vi "Add Channel Name.vi"(8 "error in (no error)":errorcluster, 9 "Channel Names":string[](array[string]), 10 "Table Name":string, 11 "Abstruct Data Type in":refnum<class "Abstruct Data Type.lvclass">) -> (0 "error out":errorcluster, 3 "Abstruct Data Type out":refnum<class "Abstruct Data Type.lvclass">)   [LabVIEW 2020, in "Abstruct Data Type.lvclass"]
uses:
  Abstruct Data Type.lvclass
  Abstruct Data Type.lvclass/Abstruct Data Type.ctl
  Data List/Data List.lvclass/Data List.ctl
  Data List/Data List.lvclass
  Data List/Accessors/Read Table Name.vi
  2984df62-0dc3-48fe-846c-8cf793447fad.vi
  Data List/Accessors/Write Table Name.vi
  Data List/Accessors/Write Channels Names.vi
  Data List/Accessors/Write File Path.vi
  Data List/Accessors/Read Channels Names.vi
  Accessors/Read Table Infor.vi
  Accessors/Read File Path.vi
  Accessors/Write Table Infor.vi
  2984df62-0dc3-48fe-846c-8cf793447fad.vi/d4db2432-cc9c-482c-8957-dac855435ef6.vi
  2984df62-0dc3-48fe-846c-8cf793447fad.vi/86fbf154-bd7b-49a2-8ab2-a837b2a95f24.vi
  2984df62-0dc3-48fe-846c-8cf793447fad.vi/3b95b01e-1ec2-4565-bcd9-7606a5281010.vi
  2984df62-0dc3-48fe-846c-8cf793447fad.vi/96a08935-737a-44b2-979c-a81d56408f7e.vi
  2984df62-0dc3-48fe-846c-8cf793447fad.vi/d4db2432-cc9c-482c-8957-dac855435ef6.vi/6eaecd13-6e48-4772-a921-b51ebdf84d88.vi
  2984df62-0dc3-48fe-846c-8cf793447fad.vi/d4db2432-cc9c-482c-8957-dac855435ef6.vi/d2d5f2b7-06f4-47f6-971c-049c3fdbb653.vi
  2984df62-0dc3-48fe-846c-8cf793447fad.vi/3b95b01e-1ec2-4565-bcd9-7606a5281010.vi/6eaecd13-6e48-4772-a921-b51ebdf84d88.vi
  2984df62-0dc3-48fe-846c-8cf793447fad.vi/3b95b01e-1ec2-4565-bcd9-7606a5281010.vi/d2d5f2b7-06f4-47f6-971c-049c3fdbb653.vi
  2984df62-0dc3-48fe-846c-8cf793447fad.vi/96a08935-737a-44b2-979c-a81d56408f7e.vi/6eaecd13-6e48-4772-a921-b51ebdf84d88.vi
  2984df62-0dc3-48fe-846c-8cf793447fad.vi/96a08935-737a-44b2-979c-a81d56408f7e.vi/d2d5f2b7-06f4-47f6-971c-049c3fdbb653.vi
  <vilib>/Comparison/Less/Less Functor/Less Functor.lvclass
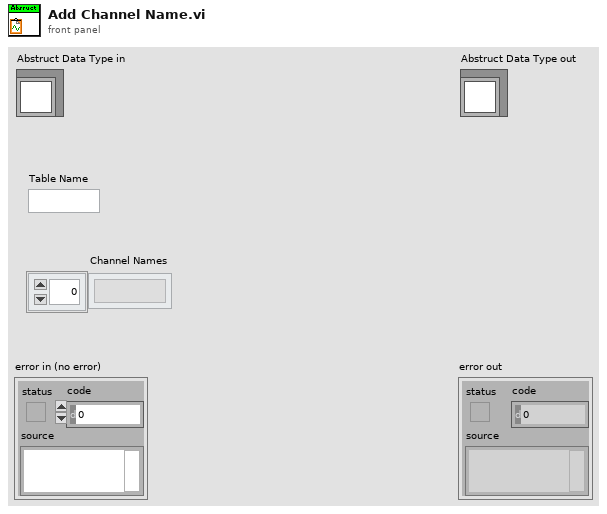
[diagram p1: front panel]
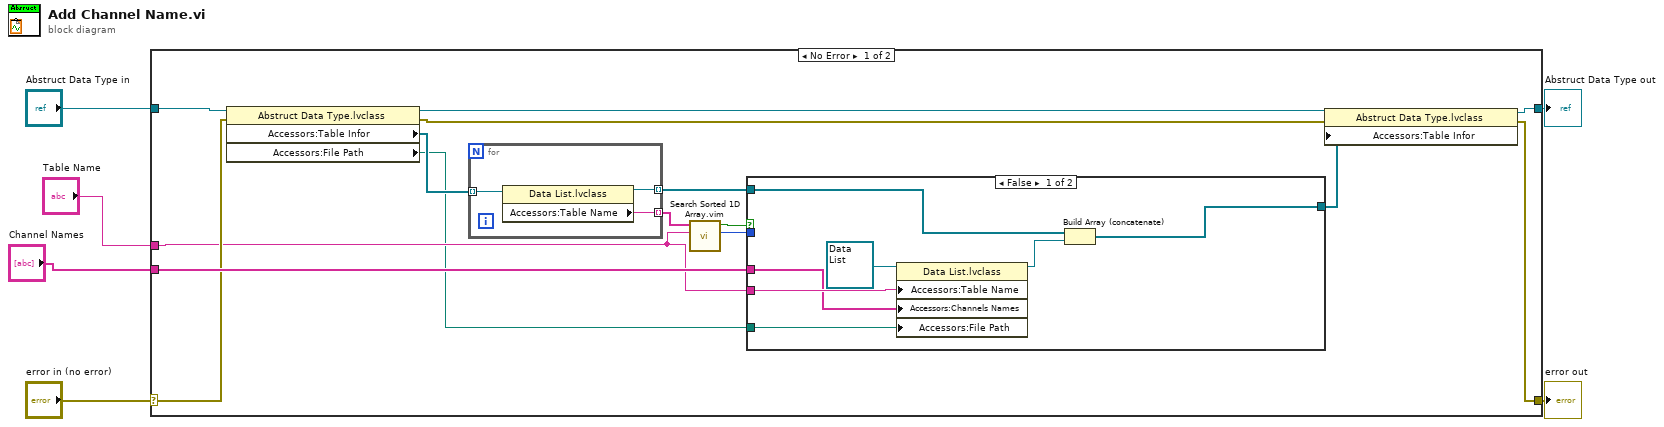
[diagram p0: block diagram]
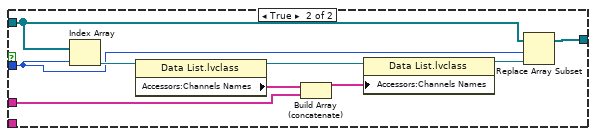
[diagram p2: hidden frame]
diagram:
  n1 = case shown="No Error" "error in (no error)" {
    selector: "error in (no error)" -> [w9 w42]
    tunnel: [w11 w42] -> w5
    tunnel: [w12 w41] -> w3
    tunnel: "Abstruct Data Type in" -> [w21 w41]
    tunnel: "Table Name" -> [w8 _]
    tunnel: "Channel Names" -> [w15 _]
    frame No Error {
      n2 = property class="Abstruct Data Type.lvclass"(reference=w21, error in=w9) -> (reference out=w13:refnum<class "Abstruct Data Type.lvclass">, error out=w10:errorcluster, "Accessors:Table Infor"=w20:refnum<class "Data List.lvclass">[], "Accessors:File Path"=w7:path)
      n3 = for {
        tunnel: w20 -> [w40] mode=indexing
        tunnel: [w39] -> w16 mode=indexing
        tunnel: [w38] -> w19 mode=indexing
        n4 = property class="Data List.lvclass"(reference=w40) -> (reference out=w39:refnum<class "Data List.lvclass">, "Accessors:Table Name"=w38:string)  [unwired: 1 in, 1 out]
      }
      n5 = call "Search Sorted 1D Array.vim"("element"=w8, "sorted 1D array"=w19) -> ("nearest index"=w17:i32, "found?"=w18:bool)  [unwired: 8 in]
      n6 = case shown="False" w18 {
        tunnel: w17 -> [_ w31]
        tunnel: w16 -> [w28 w32]
        tunnel: w15 -> [w23 w34]
        tunnel: [w25 w29] -> w14
        tunnel: w8 -> [w24 _]
        tunnel: w7 -> [w22 _]
        frame False {
          n7 = property class="Data List.lvclass"(reference=refnum<class "Data List.lvclass"> refnum ("Data List.lvclass"), "Accessors:Table Name"=w24, "Accessors:Channels Names"=w23, "Accessors:File Path"=w22) -> (reference out=w26:refnum<class "Data List.lvclass">)  [unwired: 1 in, 1 out]
          n8 = Build Array (concatenate)(w28, w26) -> (w25:refnum<class "Data List.lvclass">[])
        }
        frame True {
          n9 = Index Array(array=w32, index=w31) -> (element=w37:refnum<class "Data List.lvclass">)
          n10 = property class="Data List.lvclass"(reference=w37) -> (reference out=w33:refnum<class "Data List.lvclass">, "Accessors:Channels Names"=w36:string[])  [unwired: 1 in, 1 out]
          n11 = Build Array (concatenate)(w36, w34) -> (w35:string[])
          n12 = property class="Data List.lvclass"(reference=w33, "Accessors:Channels Names"=w35) -> (reference out=w30:refnum<class "Data List.lvclass">)  [unwired: 1 in, 1 out]
          n13 = Replace Array Subset(array=w32, new element=w30, index=w31) -> (w29:refnum<class "Data List.lvclass">[])
        }
      }
      n14 = property class="Abstruct Data Type.lvclass"(reference=w13, error in=w10, "Accessors:Table Infor"=w14) -> (reference out=w12:refnum<class "Abstruct Data Type.lvclass">, error out=w11:errorcluster)
    }
    frame Error {
    }
  }
  "error out" <- w5
  "Abstruct Data Type out" <- w3
